vi "Model - Init.vi"(8 "error in (no error)":errorcluster) -> (0 "error out":errorcluster, 3 "View Model":T1)   [LabVIEW 2017]
uses:
  Controls/View Model.ctl
  Configuration Database/Controls/Config Model.ctl
  Configuration Database/Controls/Config Commands.ctl
  Configuration Database/Controls/Congif Data.ctl
  Controls/Shared Model.ctl
  Error Handler/Controls/Error Model.ctl
  Error Handler/Controls/Error Data.ctl
  Error Handler/Controls/Error Type.ctl
  Car Wash Controller/Controls/Car Wash Model.ctl
  Car Wash Controller/Controls/Controller Overhead.ctl
  Car Wash Controller/Controls/Vehicle Location.ctl
  Car Wash Controller/Controls/Car Wash States.ctl
  Car Wash Controller/Controls/CarWash CMD.ctl
  Views/Wash Display Console View/Controls/Car Wash Indicators.ctl
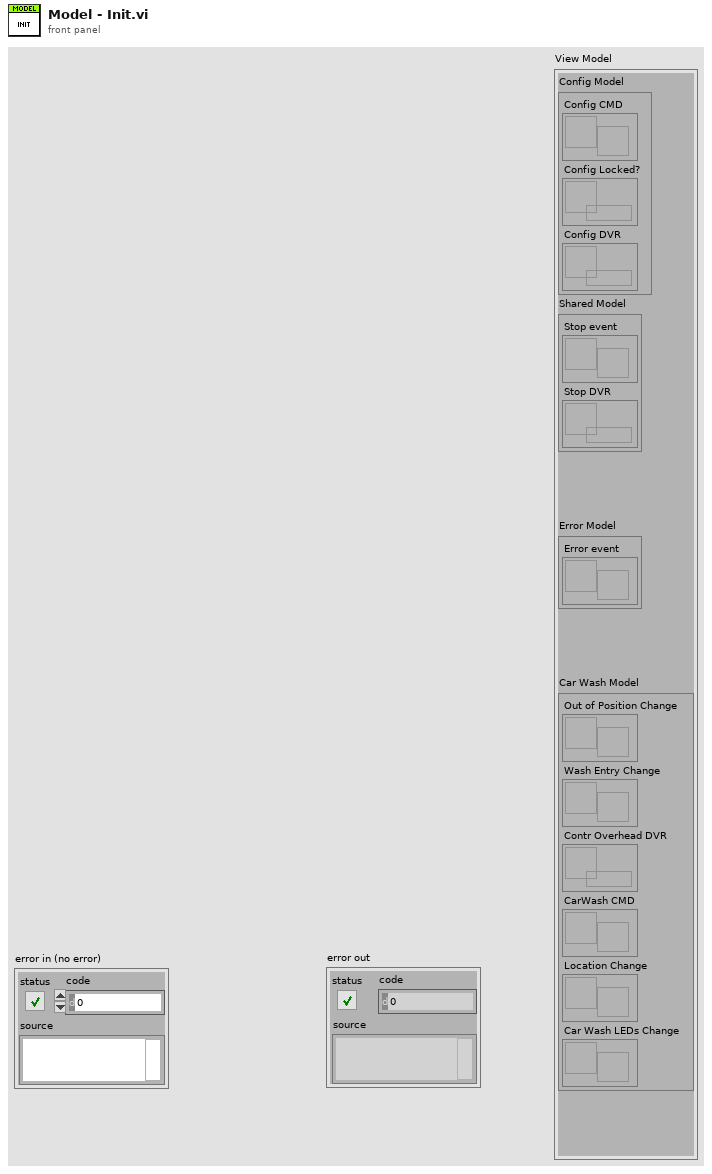
[diagram p1: front panel]
types:
  T1 = typedef "View Model.ctl" = cluster{"Config Model":T2, "Shared Model":T3, "Error Model":T4, "Car Wash Model":T5}
  T2 = typedef "Config Model.ctl" = cluster{"Config CMD":refnum<user-event>, "Config Locked?":refnum<data-value>, "Config DVR":refnum<data-value>}
  T3 = typedef "Shared Model.ctl" = cluster{"Stop event":refnum<user-event>, "Stop DVR":refnum<data-value>}
  T4 = typedef "Error Model.ctl" = cluster{"Error event":refnum<user-event>}
  T5 = typedef "Car Wash Model.ctl" = cluster{"Out of Position Change":refnum<user-event>, "Wash Entry Change":refnum<user-event>, "Contr Overhead DVR":refnum<data-value>, "CarWash CMD":refnum<user-event>, "Location Change":refnum<user-event>, "Car Wash LEDs Change":refnum<user-event>}
  T6 = typedef "Car Wash Indicators.ctl" = cluster{"Under Body Wash":bool, "Bug Remover":bool, "Pre-Soak":bool, "High Pressure Wash":bool, "Low Pressure Wax":bool, "Spot Free Rinse":bool, "Tire Shine Foam":bool, "Air Dry":bool}
  T7 = typedef "Vehicle Location.ctl" = enum16{"Entry", "Station 1", "Station 2", "Station 3", "Exit"}
  T8 = typedef "CarWash CMD.ctl" = cluster{"CarWash States":T9, "Variant":variant}
  T9 = typedef "Car Wash States.ctl" = enum16{"Initial", "Wait for start", "Start", "Wait for vehicle", "Wash Step Execution", "Wash Step/Cycle Complete", "Wash Exit", "Wash Abort/Terminate"}
  T10 = typedef "Controller Overhead.ctl" = cluster{"Location change":bool, "Vehicle Location":T7, "CarWash State":T9, "CarWash Next State":T9, "Start change":bool, "Time":dbl, "Elapsed Time":dbl}
  T11 = typedef "Error Data.ctl" = cluster{"Error Type":T12, "Error cluster":errorcluster, "Other Data":variant}
  T12 = typedef "Error Type.ctl" = enum16{"Minor Error", "Wash Cycle Error", "System Error", "Other Error"}
  T13 = typedef "Congif Data.ctl" = cluster{"Wash Step":string, "Station":string, "Step Duration":u32}
  T14 = typedef "Config Commands.ctl" = enum16{"Read records", "Query timing data", "Insert new data records", "Update data records"}
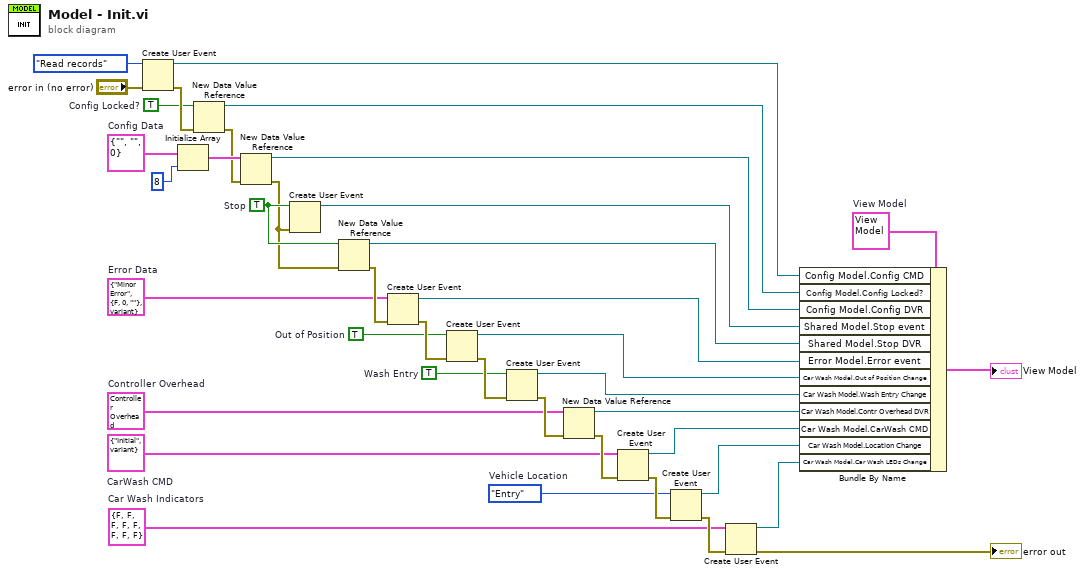
[diagram p0: block diagram]
diagram:
  w4 = T6 {"Under Body Wash"=FALSE, "Bug Remover"=FALSE, "Pre-Soak"=FALSE, "High Pressure Wash"=FALSE, "Low Pressure Wax"=FALSE, "Spot Free Rinse"=FALSE, "Tire Shine Foam"=FALSE, "Air Dry"=FALSE}  # Car Wash Indicators
  w7 = Vehicle_Location."Entry"  # Vehicle Location
  w10 = T8 {"CarWash States"=enum."Initial", "Variant"=variant}  # CarWash CMD
  w15 = TRUE  # Wash Entry
  w18 = TRUE  # Out of Position
  w13 = T10 {"Location change"=FALSE, "Vehicle Location"=enum."Entry", "CarWash State"=enum."Initial", "CarWash Next State"=enum."Initial", "Start change"=FALSE, "Time"=0.0, "Elapsed Time"=0.0}  # Controller Overhead
  w22 = T11 {"Error Type"=enum."Minor Error", "Error cluster"={"status"=FALSE, "code"=0, "source"=""}, "Other Data"=variant}  # Error Data
  w26 = TRUE  # Stop
  w35 = TRUE  # Config Locked?
  w33 = T13 {"Wash Step"="", "Station"="", "Step Duration"=0}  # Config Data
  w39 = T1 {"Config Model"={"Config CMD"=refnum, "Config Locked?"=refnum, "Config DVR"=refnum}, "Shared Model"={"Stop event"=refnum, "Stop DVR"=refnum}, "Error Model"={"Error event"=refnum}, "Car Wash Model"={"Out of Position Change"=refnum, "Wash Entry Change"=refnum, "Contr Overhead DVR"=refnum, "CarWash CMD"=refnum, "Location Change"=refnum, "Car Wash LEDs Change"=refnum}}  # View Model
  n1 = Create User Event(user event datatype=Config_Commands."Read records" ("Config Command"), error in="error in (no error)") -> (user event=w37:refnum<user-event>, error out=w36:errorcluster)
  n2 = Initialize Array(w33, 8 ("dimension size")) -> (w31:T13[])
  n3 = New Data Value Reference(data value=w35, error in=w36) -> (data value reference=w34:refnum<data-value>, error out=w30:errorcluster)
  n4 = New Data Value Reference(data value=w31, error in=w30) -> (data value reference=w29:refnum<data-value>, error out=w25:errorcluster)
  n5 = Create User Event(user event datatype=w26, error in=w25) -> (user event=w27:refnum<user-event>)  [unwired: 1 out]
  n6 = New Data Value Reference(data value=w26, error in=w25) -> (data value reference=w24:refnum<data-value>, error out=w23:errorcluster)
  n7 = Create User Event(user event datatype=w22, error in=w23) -> (user event=w21:refnum<user-event>, error out=w20:errorcluster)
  n8 = Create User Event(user event datatype=w18, error in=w20) -> (user event=w17:refnum<user-event>, error out=w19:errorcluster)
  n9 = Create User Event(user event datatype=w15, error in=w19) -> (user event=w16:refnum<user-event>, error out=w14:errorcluster)
  n10 = New Data Value Reference(data value=w13, error in=w14) -> (data value reference=w12:refnum<data-value>, error out=w11:errorcluster)
  n11 = Create User Event(user event datatype=w10, error in=w11) -> (user event=w9:refnum<user-event>, error out=w8:errorcluster)
  n12 = Create User Event(user event datatype=w7, error in=w8) -> (user event=w6:refnum<user-event>, error out=w5:errorcluster)
  n13 = Create User Event(user event datatype=w4, error in=w5) -> (user event=w3:refnum<user-event>, error out=→"error out":errorcluster)
  n14 = Bundle By Name(cluster=w39, "Config Model.Config CMD"=w37, "Config Model.Config Locked?"=w34, "Config Model.Config DVR"=w29, "Shared Model.Stop event"=w27, "Shared Model.Stop DVR"=w24, "Error Model.Error event"=w21, "Car Wash Model.Out of Position Change"=w17, "Car Wash Model.Wash Entry Change"=w16, "Car Wash Model.Contr Overhead DVR"=w12, "Car Wash Model.CarWash CMD"=w9, "Car Wash Model.Location Change"=w6, "Car Wash Model.Car Wash LEDs Change"=w3) -> (→"View Model":T1)
